vi "Set Bool Green.vi"(8 "error in (no error)":errorcluster, 11 "Indicator ref in":refnum<vi>) -> (0 "error out":errorcluster)   [LabVIEW 2024]
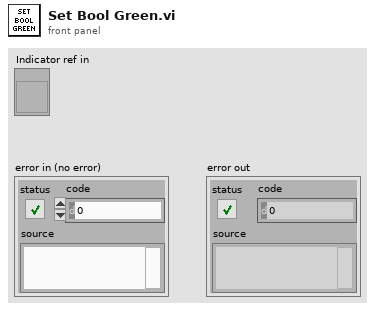
[diagram p1: front panel]
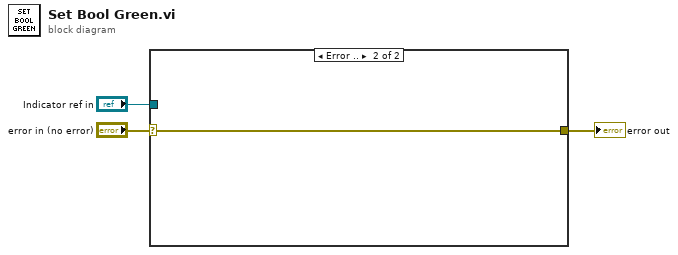
[diagram p0: block diagram]
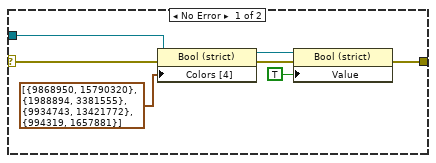
[diagram p2: hidden frame]
diagram:
  n1 = case shown="Error .." "error in (no error)" {
    selector: "error in (no error)" -> [w4 w11]
    tunnel: "Indicator ref in" -> [w7 _]
    tunnel: [w5 w11] -> w2
    frame No Error {
      n2 = property class="Bool (strict)"(reference=w7, error in=w4, "Colors [4]"=cluster{u32, u32}[] [{9868950, 15790320}, {1988894, 3381555}, {9934743, 13421772}, {994319, 1657881}]) -> (reference out=w10:refnum<vi>, error out=w9:errorcluster)
      n3 = property class="Bool (strict)"(reference=w10, error in=w9, "Value"=TRUE) -> (error out=w5:errorcluster)  [unwired: 1 out]
    }
    frame Error {
    }
  }
  "error out" <- w2
